vi "Close Real ActiveX Reference.vi"(8 "error in (no error)":errorcluster, 11 "Generic ActiveX":refnum<k7>) -> (0 "error out":errorcluster)   [LabVIEW 2017]
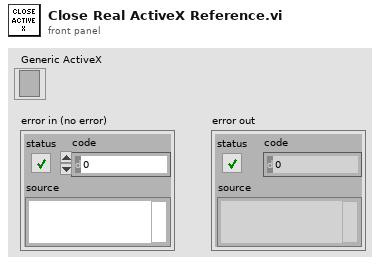
[diagram p1: front panel]
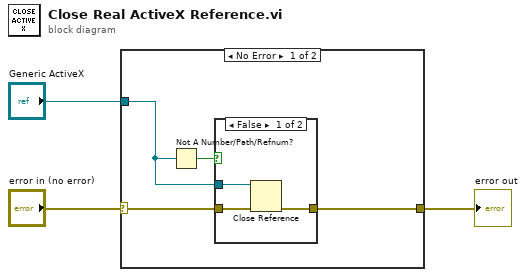
[diagram p0: block diagram]
diagram:
  n1 = case shown="No Error" "error in (no error)" {
    selector: "error in (no error)" -> [w7 w12]
    tunnel: "Generic ActiveX" -> [w5 _]
    tunnel: [w6 w12] -> w1
    frame No Error {
      n2 = Not A Number/Path/Refnum?(number/path/refnum=w5) -> (NaN/Path/Refnum?=w4:bool)
      n3 = case shown="False" w4 {
        tunnel: w7 -> [w10 w11]
        tunnel: [w9 w11] -> w6
        tunnel: w5 -> [w8 _]
        frame False {
          n4 = Close Reference(reference=w8, error in (no error)=w10) -> (error out=w9:errorcluster)
        }
        frame True {
        }
      }
    }
    frame Error {
    }
  }
  "error out" <- w1
